vi "SetGlobalVariables.vi"   [LabVIEW 2020]
doc: "This VI sets non-robot specific constants and initializes critical global variables."
uses:
  GlobalMiscellaneous.vi
  GlobalDrivebase.vi
  GlobalPoseAndTargeting.vi
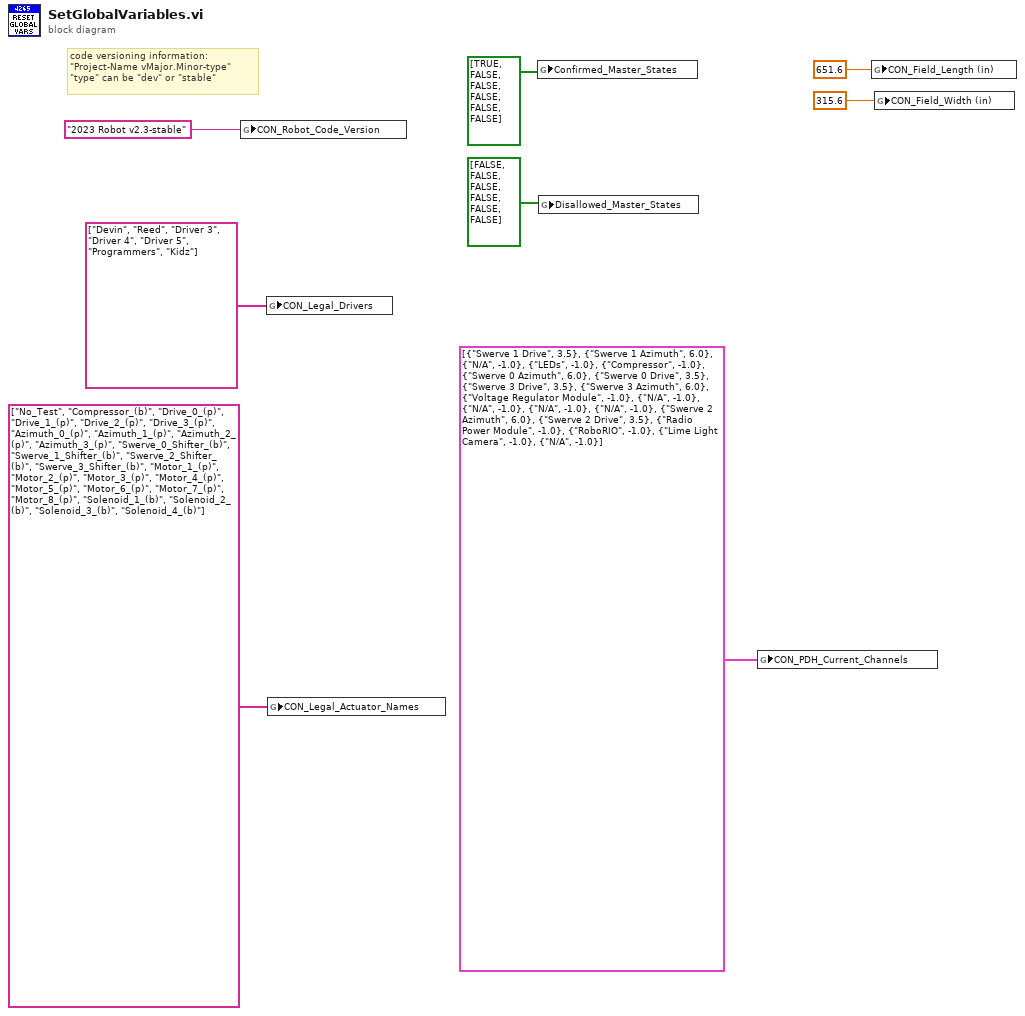
[diagram p0: block diagram]
diagram:
  # "code versioning information:\n\"Project-Name vMajor.Minor-type\"\n\"type\" can be \"dev\" or \"stable\""
  n1 = global write "GlobalMiscellaneous.vi" "CON_Robot_Code_Version"("2023 Robot v2.3-stable" ("CON_Robot_Code_Version")) -> ()
  n2 = global write "GlobalDrivebase.vi" "CON_Legal_Drivers"(string[] ["Devin", "Reed", "Driver 3", "Driver 4", "Driver 5", "Programmers", "Kidz"] ("appended array")) -> ()
  n3 = global write "GlobalMiscellaneous.vi" "CON_Legal_Actuator_Names"(string[] ["No_Test", "Compressor_(b)", "Drive_0_(p)", "Drive_1_(p)", "Drive_2_(p)", "Drive_3_(p)", "Azimuth_0_(p)", "Azimuth_1_(p)", "Azimuth_2_(p)", "Azimuth_3_(p)", "Swerve_0_Shifter_(b)", "Swerve_1_Shifter_(b)", "Swerve_2_Shifter_(b)", "Swerve_3_Shifter_(b)", "Motor_1_(p)", "Motor_2_(p)", "Motor_3_(p)", "Motor_4_(p)", "Motor_5_(p)", "Motor_6_(p)", "Motor_7_(p)", "Motor_8_(p)", "Solenoid_1_(b)", "Solenoid_2_(b)", "Solenoid_3_(b)", "Solenoid_4_(b)"] ("appended array")) -> ()
  n4 = global write "GlobalMiscellaneous.vi" "Confirmed_Master_States"(bool[] [TRUE, FALSE, FALSE, FALSE, FALSE, FALSE] ("Disallowed_Master_States")) -> ()
  n5 = global write "GlobalMiscellaneous.vi" "Disallowed_Master_States"(bool[] [FALSE, FALSE, FALSE, FALSE, FALSE, FALSE] ("Disallowed_Master_States")) -> ()
  n6 = global write "GlobalMiscellaneous.vi" "CON_PDH_Current_Channels"(cluster{string, dbl}[] [{"Swerve 1 Drive", 3.5}, {"Swerve 1 Azimuth", 6.0}, {"N/A", -1.0}, {"LEDs", -1.0}, {"Compressor", -1.0}, {"Swerve 0 Azimuth", 6.0}, {"Swerve 0 Drive", 3.5}, {"Swerve 3 Drive", 3.5}, {"Swerve 3 Azimuth", 6.0}, {"Voltage Regulator Module", -1.0}, {"N/A", -1.0}, {"N/A", -1.0}, {"N/A", -1.0}, {"N/A", -1.0}, {"Swerve 2 Azimuth", 6.0}, {"Swerve 2 Drive", 3.5}, {"Radio Power Module", -1.0}, {"RoboRIO", -1.0}, {"Lime Light Camera", -1.0}, {"N/A", -1.0}]) -> ()
  n7 = global write "GlobalPoseAndTargeting.vi" "CON_Field_Length (in)"(651.6 ("CON_Field_Length (in)")) -> ()
  n8 = global write "GlobalPoseAndTargeting.vi" "CON_Field_Width (in)"(315.6 ("CON_Field_Length (in)")) -> ()
